vi "File Save RPM.vi"(8 "error in (no error)":errorcluster, 10 "XY Graph":cluster{"X":dbl, "Y":dbl}[](array[cluster]), 11 "File Name":path) -> (0 "error out":errorcluster)   [LabVIEW 2017]
doc: "This VI saves the RPM graph into CSV.\n\nThe RPM graph is already in an XY format so I didn't have to do some conversion. I just have to extract the data from the waveform."
uses:
  <vilib>/Utility/file.llb/Write Delimited Spreadsheet (string).vi
  <vilib>/Utility/file.llb/Write Delimited Spreadsheet (DBL).vi
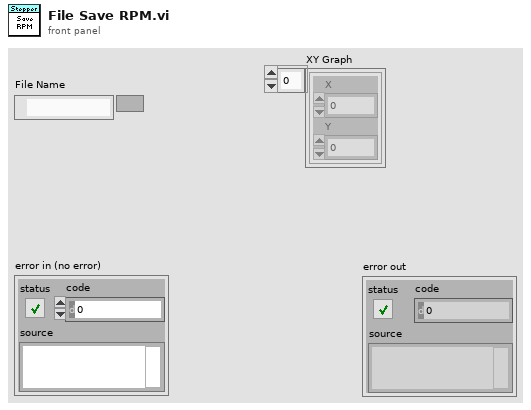
[diagram p1: front panel]
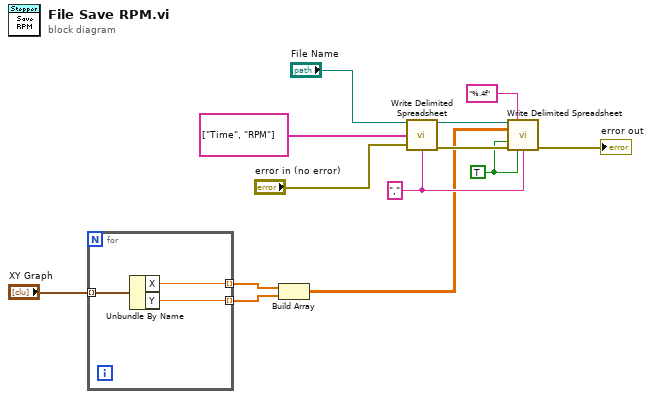
[diagram p0: block diagram]
diagram:
  w11 = TRUE ("append to file? (new file:F)")
  w10 = "," ("delimiter (\\t)")
  n1 = for {
    tunnel: "XY Graph" -> [w16] mode=indexing
    tunnel: [w15] -> w3 mode=indexing
    tunnel: [w14] -> w2 mode=indexing
    n2 = Unbundle By Name(w16) -> ("X"=w15:dbl, "Y"=w14:dbl)
  }
  n3 = Build Array(w3, w2) -> (w1:dbl[][])
  n4 = call-poly <vilib>:"Write Delimited Spreadsheet.vi"("file path (dialog if empty)"="File Name", "1D data"=string[] ["Time", "RPM"], "error in (no error)"="error in (no error)", "delimiter (\\t)"=w10) -> ("new file path (Not A Path if cancelled)"=w13:path, "error out"=w12:errorcluster)  [unwired: 10 in]
  n5 = call-poly <vilib>:"Write Delimited Spreadsheet.vi"("file path (dialog if empty)"=w13, "format (%.3f)"="%.4f", "2D data"=w1, "append to file? (new file:F)"=w11, "error in (no error)"=w12, "transpose? (no:F)"=w11, "delimiter (\\t)"=w10) -> ("error out"=→"error out":errorcluster)  [unwired: 7 in, 1 out]
